vi "Get Ref Clock Source.vi"(8 "error in (no error)":errorcluster, 11 "VISA resource name":refnum<visa-resource-name>) -> (0 "error out":errorcluster, 2 "Reference Source":u16, 3 "VISA resource name out":refnum<visa-resource-name>)   [LabVIEW 2013, in "Fluke 5XXX Series Multicalibrators.lvlib"]
doc: "This VI returns the reference clock source (internal or through the 10 MHz IN BNC connector).\n\nNote:\n\nThis VI is available only for instrument model 5520A."
uses:
  Fluke 5XXX Series Multicalibrators.lvlib
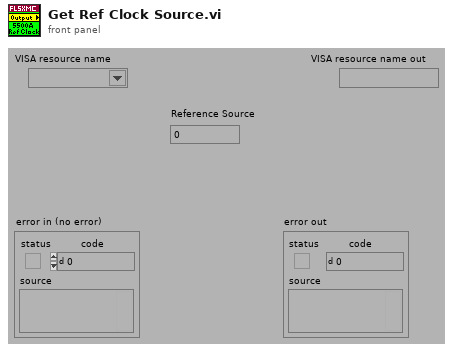
[diagram p1: front panel]
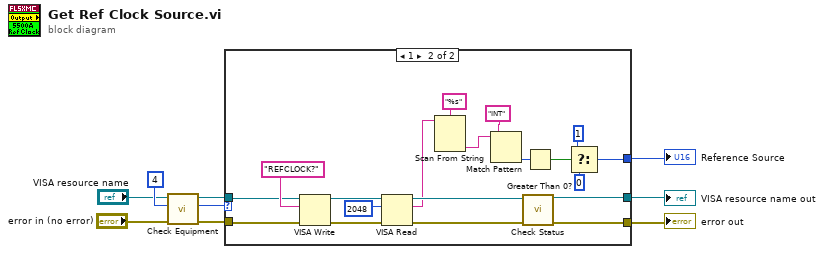
[diagram p0: block diagram]
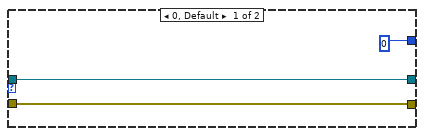
[diagram p2: hidden frame]
diagram:
  n1 = call "Check Equipment.vi"("error in (no error)"="error in (no error)", "Bit Mask"=4 ("Numeric"), "VISA resource name"="VISA resource name") -> ("error out"=w8:errorcluster, "Present?"=w7:u32, "VISA resource name out"=w6:refnum<visa-resource-name>)  [unwired: 6 in]
  n2 = case shown="1" w7 {
    tunnel: [w11 w25] -> w3
    tunnel: [w10 w22] -> w4
    tunnel: w8 -> [w11 w27]
    tunnel: w6 -> [w10 w26]
    tunnel: [u16 0 w13] -> w5
    frame 0, Default {
    }
    frame 1 {
      n3 = VISA Write(VISA resource name=w26, write buffer="REFCLOCK?", error in (no error)=w27) -> (VISA resource name out=w30:refnum<visa-resource-name>, error out=w29:errorcluster)  [unwired: 1 out]
      n4 = VISA Read(VISA resource name=w30, byte count=u32 2048 ("byte count (0)"), error in (no error)=w29) -> (VISA resource name out=w23:refnum<visa-resource-name>, read buffer=w15:string, error out=w24:errorcluster)  [unwired: 1 out]
      n5 = Scan From String(format string="%s", input string=w15) -> (output 1=w14:string)  [unwired: 3 in, 3 out]
      n6 = Match Pattern(string=w14, regular expression="INT") -> (offset past match=w19:i32)  [unwired: 1 in, 3 out]
      n7 = call "Check Status.vi"("VISA resource name"=w23, "error in (no error)"=w24) -> ("VISA resource name out"=w22:refnum<visa-resource-name>, "error out"=w25:errorcluster)  [unwired: 12 in]
      n8 = Greater Than 0?(x=w19) -> (x > 0?=w16:bool)
      n9 = Select(t=u16 1 ("f"), s=w16, f=u16 0) -> (s? t:f=w13:u16)
    }
  }
  "Reference Source" <- w5
  "VISA resource name out" <- w4
  "error out" <- w3
